vi "solar_write LogRestart.vi"(8 "error in (no error)":errorcluster, 10 "Restart":bool=TRUE, 11 "solar in":refnum<class "solar.lvclass">) -> (0 "error out":errorcluster, 3 "solar out":refnum<class "solar.lvclass">)   [LabVIEW 2018, in "solar.lvclass"]
doc: "If true, this restart the solar log file."
uses:
  solar.lvclass
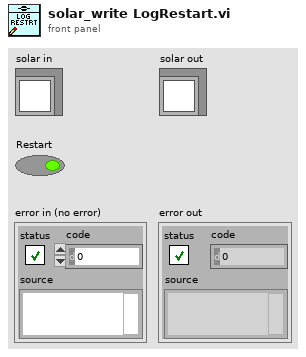
[diagram p1: front panel]
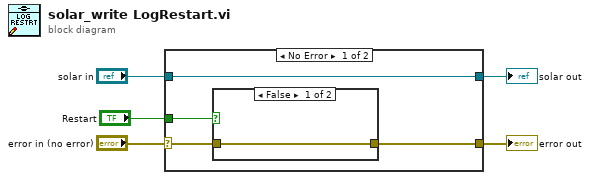
[diagram p0: block diagram]
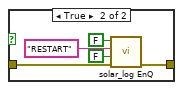
[diagram p2: hidden frame]
diagram:
  n1 = case shown="No Error" "error in (no error)" {
    selector: "error in (no error)" -> [w8 w17]
    tunnel: "solar in" -> [w9 w16]
    tunnel: [w7 w17] -> w4
    tunnel: [w9 w16] -> w2
    tunnel: "Restart" -> [w6 _]
    frame No Error {
      n2 = case shown="False" w6 {
        tunnel: w8 -> [w10 w12]
        tunnel: [w10 w11] -> w7
        frame False {
        }
        frame True {
          n3 = call "solar_log EnQ.vi"("error in (no error)"=w12, "Front? (F)"=FALSE, "MSG"="RESTART", "Create? (F)"=FALSE) -> ("error out"=w11:errorcluster)  [unwired: 5 in, 2 out]
        }
      }
    }
    frame Error {
    }
  }
  "error out" <- w4
  "solar out" <- w2
